vi "bin_without_level_with_enable_final.vi"() -> ()   [LabVIEW 2022 SP3]
uses:
  <vilib>/DAQmx/read.llb/DAQmx Read (Analog DBL 1Chan 1Samp).vi
  <vilib>/DAQmx/read.llb/DAQmx Read (Digital Bool 1Line 1Point).vi
  <vilib>/DAQmx/write.llb/DAQmx Write (Digital Bool 1Line 1Point).vi
  <vilib>/DAQmx/write.llb/DAQmx Write (Analog DBL 1Chan 1Samp).vi
  <vilib>/DAQmx/create/channels.llb/DAQmx Create Channel (DO-Digital Output).vi
  <vilib>/DAQmx/create/channels.llb/DAQmx Create Channel (DI-Digital Input).vi
  <vilib>/DAQmx/create/channels.llb/DAQmx Create Channel (AI-Voltage-Basic).vi
  <vilib>/DAQmx/create/channels.llb/DAQmx Create Channel (AO-Voltage-Basic).vi
  <vilib>/DAQmx/miscellaneous.llb/DAQmx Fill In Error Info.vi
panel:
  out "Boolean":bool
  out "Numeric 3":dbl format="%#_3g"
  in  "Numeric 2":dbl
  in  "Numeric":dbl
  out "String":string
  out "Weight":dbl
  in  "Linear Actuator for Plastic":tag
  in  "Linear Actuator for Plastic":tag
  in  "Linear actuator for glass":tag
  in  "Linear actuator for glass":tag
  in  "Load cell":tag
  in  "Induction proximity Sensor":tag
  in  "Linear Actuator for metal":tag
  in  "Linear Actuator for metal":tag
  in  "Exit":bool
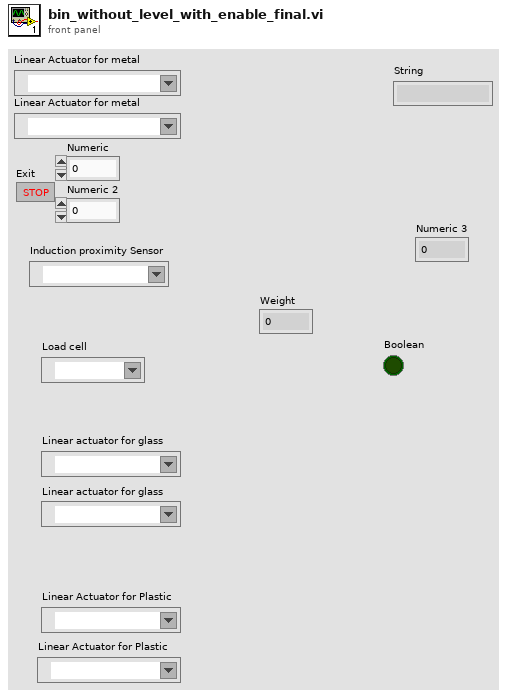
[diagram p1: front panel]
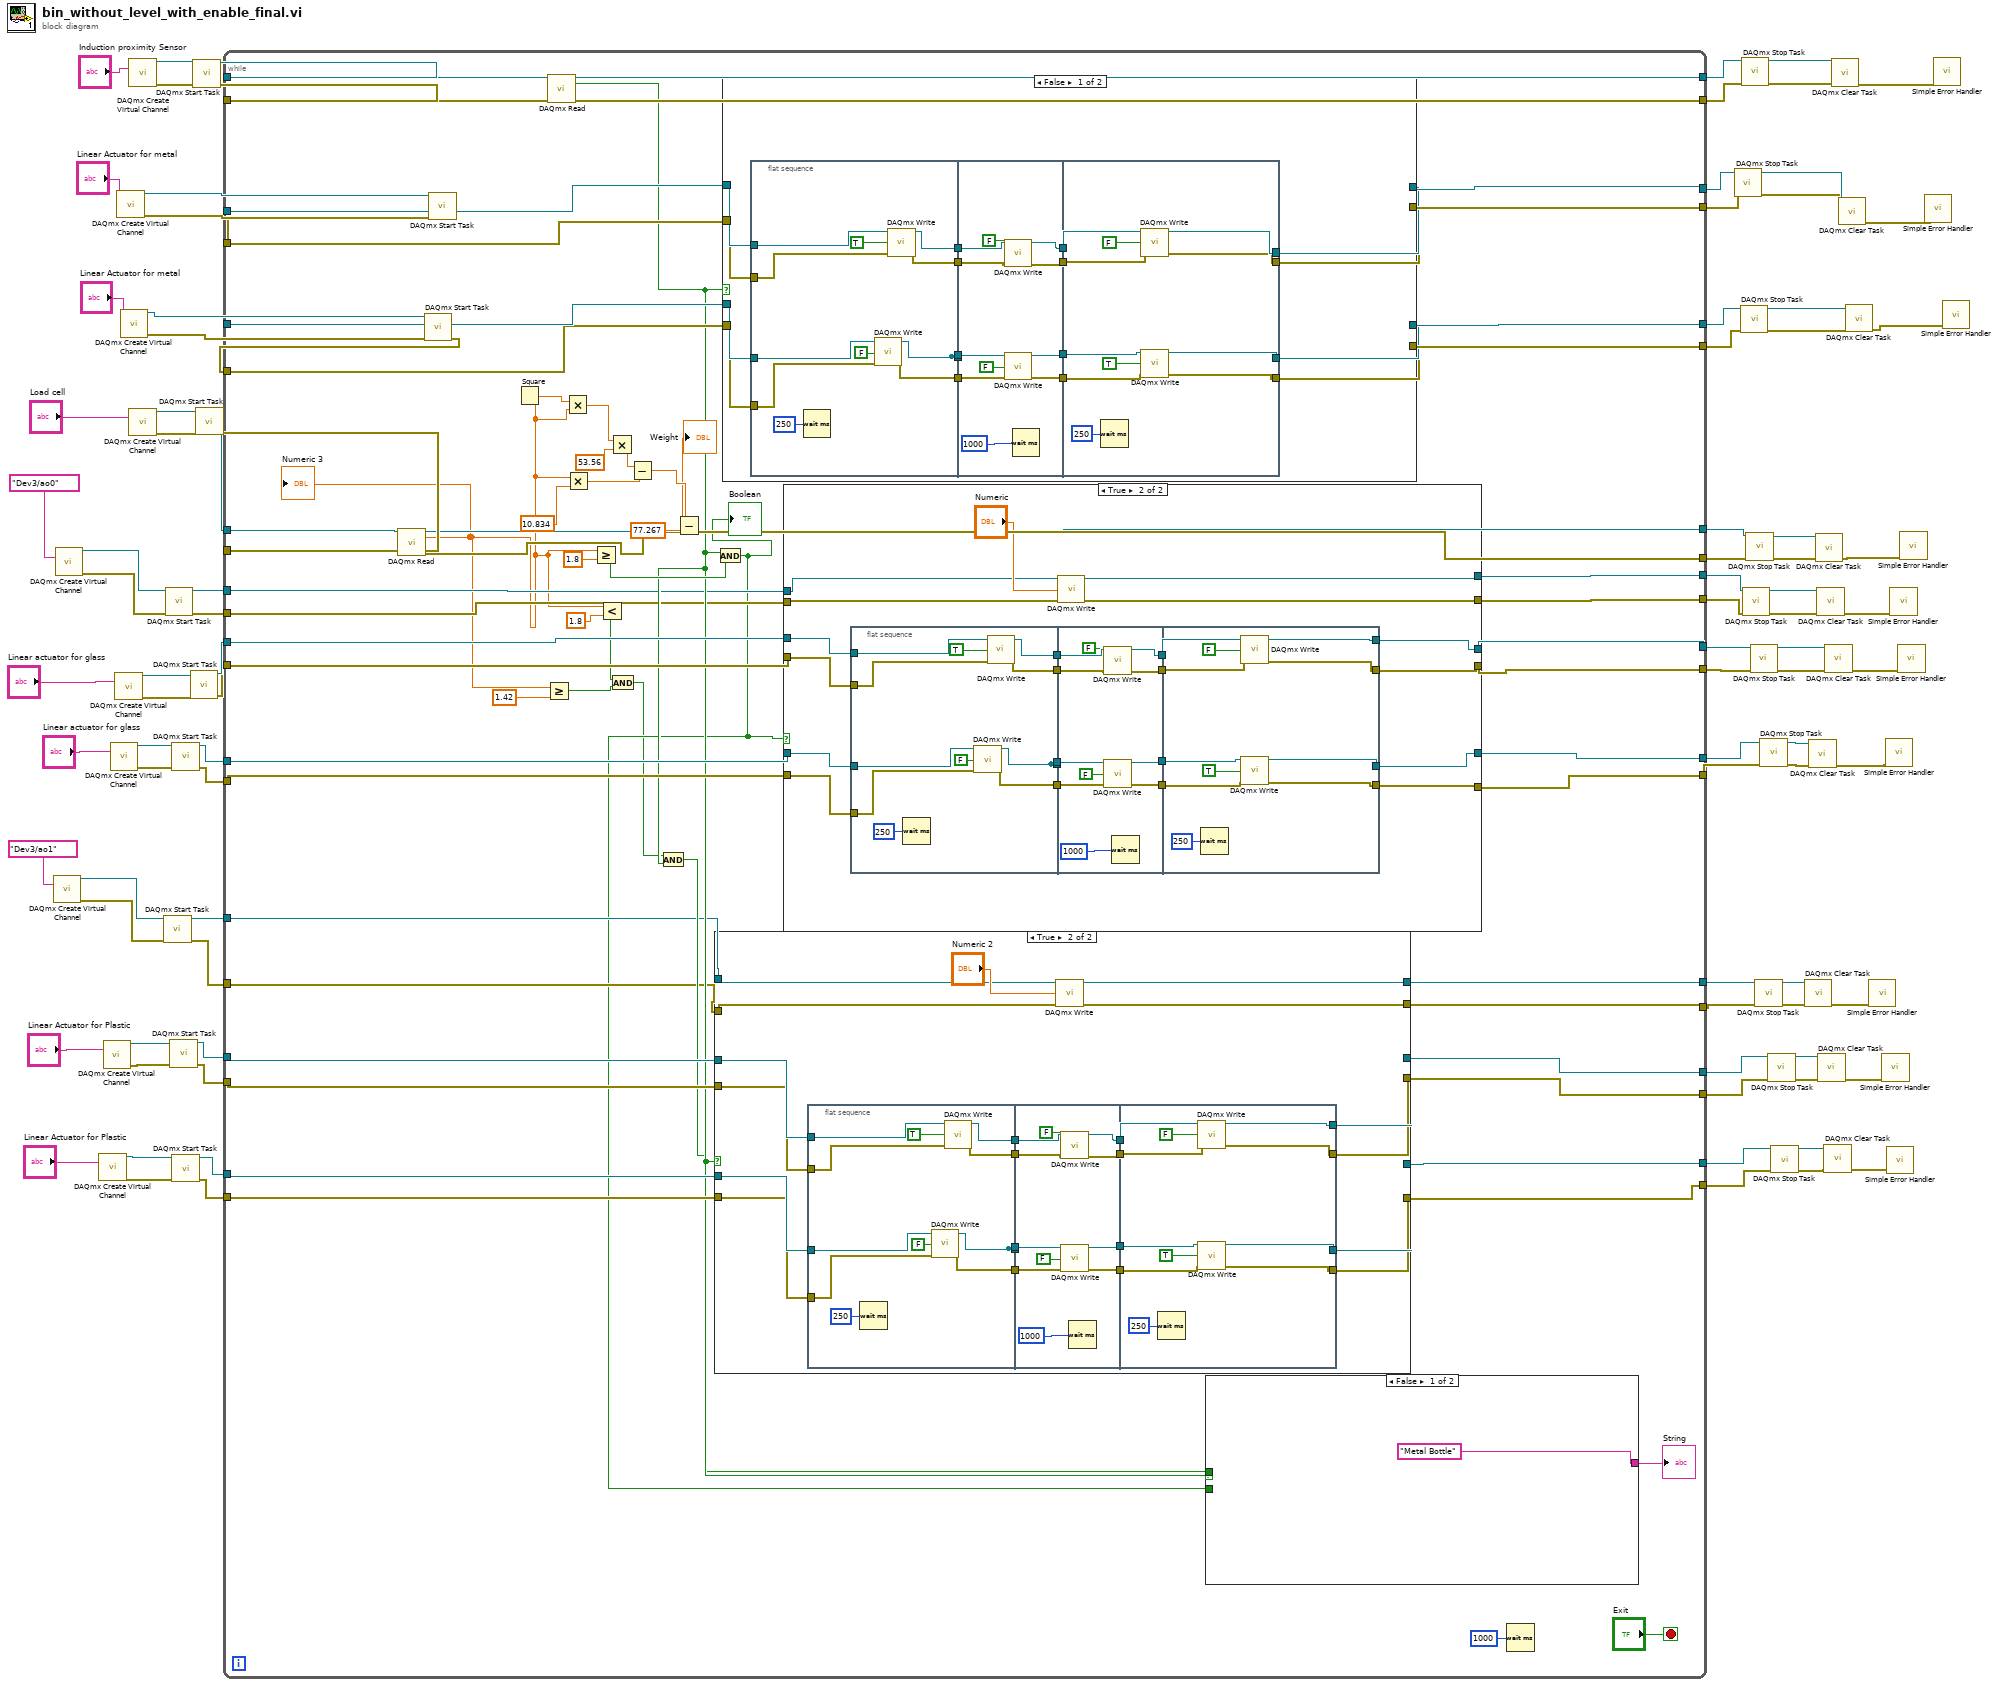
[diagram p0: block diagram]
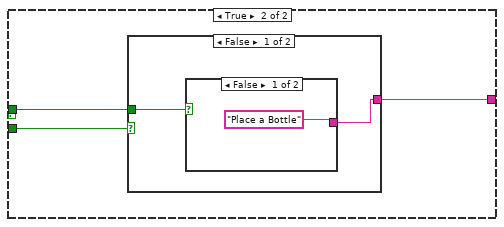
[diagram p2: hidden frame]
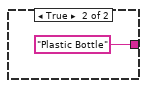
[diagram p3: hidden frame]
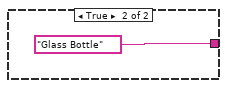
[diagram p4: hidden frame]
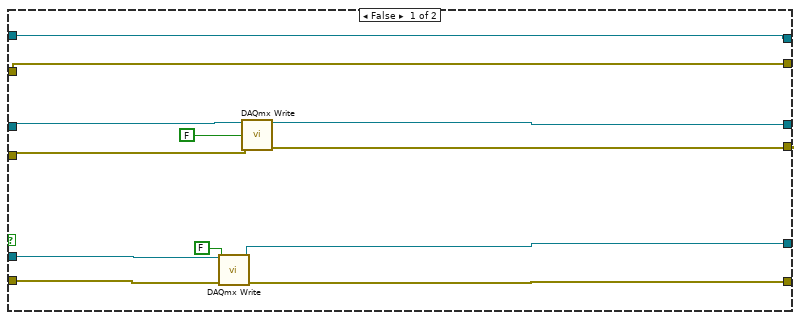
[diagram p5: hidden frame]
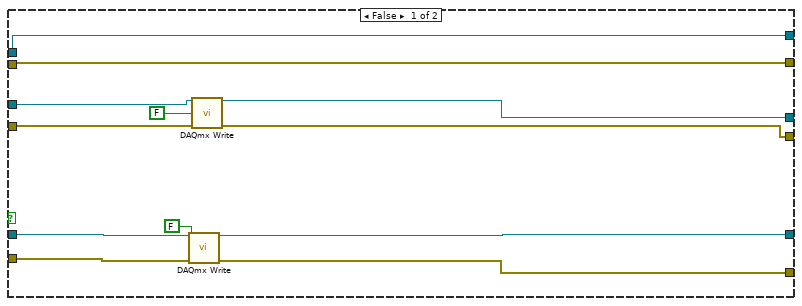
[diagram p6: hidden frame]
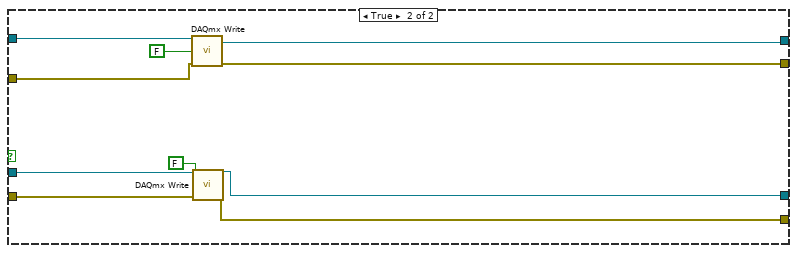
[diagram p7: hidden frame]
diagram:
  n1 = call-poly <vilib>:"DAQmx Create Virtual Channel.vi"("physical channels"=tag "Dev3/ao1") -> ("task out"=w14:refnum<k21>, "error out"=w13:errorcluster)  [unwired: 13 in]
  n2 = call-poly <vilib>:"DAQmx Create Virtual Channel.vi"("physical channels"=tag "Dev3/ao0") -> ("task out"=w19:refnum<k21>, "error out"=w18:errorcluster)  [unwired: 13 in]
  n3 = call-poly <vilib>:"DAQmx Create Virtual Channel.vi"("lines"="Linear Actuator for Plastic") -> ("task out"=w39:refnum<k21>, "error out"=w38:errorcluster)  [unwired: 13 in]
  n4 = call-poly <vilib>:"DAQmx Create Virtual Channel.vi"("lines"="Linear Actuator for Plastic") -> ("task out"=w43:refnum<k21>, "error out"=w42:errorcluster)  [unwired: 13 in]
  n5 = call-poly <vilib>:"DAQmx Create Virtual Channel.vi"("lines"="Linear actuator for glass") -> ("task out"=w59:refnum<k21>, "error out"=w58:errorcluster)  [unwired: 13 in]
  n6 = call-poly <vilib>:"DAQmx Create Virtual Channel.vi"("lines"="Linear actuator for glass") -> ("task out"=w65:refnum<k21>, "error out"=w64:errorcluster)  [unwired: 13 in]
  n7 = call-poly <vilib>:"DAQmx Create Virtual Channel.vi"("lines"="Linear Actuator for metal") -> ("task out"=w86:refnum<k21>, "error out"=w85:errorcluster)  [unwired: 13 in]
  n8 = call-poly <vilib>:"DAQmx Create Virtual Channel.vi"("lines"="Linear Actuator for metal") -> ("task out"=w90:refnum<k21>, "error out"=w89:errorcluster)  [unwired: 13 in]
  n9 = call-poly <vilib>:"DAQmx Create Virtual Channel.vi"("lines"="Induction proximity Sensor") -> ("task out"=w79:refnum<k21>, "error out"=w78:errorcluster)  [unwired: 13 in]
  n10 = call-poly <vilib>:"DAQmx Create Virtual Channel.vi"("physical channels"="Load cell") -> ("task out"=w70:refnum<k21>, "error out"=w67:errorcluster)  [unwired: 13 in]
  n11 = call <vilib>:"DAQmx Start Task.vi"("task/channels in"=w14, "error in"=w13) -> ("task out"=w12:refnum<k21>, "error out"=w11:errorcluster)  [unwired: 12 in]
  n12 = call <vilib>:"DAQmx Start Task.vi"("task/channels in"=w19, "error in"=w18) -> ("task out"=w17:refnum<k21>, "error out"=w16:errorcluster)  [unwired: 12 in]
  n13 = call <vilib>:"DAQmx Start Task.vi"("task/channels in"=w43, "error in"=w42) -> ("task out"=w41:refnum<k21>, "error out"=w40:errorcluster)  [unwired: 12 in]
  n14 = call <vilib>:"DAQmx Start Task.vi"("task/channels in"=w59, "error in"=w58) -> ("task out"=w57:refnum<k21>, "error out"=w56:errorcluster)  [unwired: 12 in]
  n15 = call <vilib>:"DAQmx Start Task.vi"("task/channels in"=w39, "error in"=w38) -> ("task out"=w37:refnum<k21>, "error out"=w36:errorcluster)  [unwired: 12 in]
  n16 = call <vilib>:"DAQmx Start Task.vi"("task/channels in"=w65, "error in"=w64) -> ("task out"=w63:refnum<k21>, "error out"=w62:errorcluster)  [unwired: 12 in]
  n17 = call <vilib>:"DAQmx Start Task.vi"("task/channels in"=w79, "error in"=w78) -> ("task out"=w77:refnum<k21>, "error out"=w76:errorcluster)  [unwired: 12 in]
  n18 = call <vilib>:"DAQmx Start Task.vi"("task/channels in"=w70, "error in"=w67) -> ("task out"=w69:refnum<k21>, "error out"=w68:errorcluster)  [unwired: 12 in]
  n19 = call <vilib>:"DAQmx Start Task.vi"("task/channels in"=w90, "error in"=w89) -> ("task out"=w88:refnum<k21>, "error out"=w87:errorcluster)  [unwired: 12 in]
  n20 = call <vilib>:"DAQmx Start Task.vi"("task/channels in"=w86, "error in"=w85) -> ("task out"=w84:refnum<k21>, "error out"=w83:errorcluster)  [unwired: 12 in]
  n21 = while {
    tunnel: w88 -> [w163]
    tunnel: w87 -> [w162]
    tunnel: w84 -> [w161]
    tunnel: w83 -> [w160]
    tunnel: [w159] -> w98
    tunnel: [w158] -> w97
    tunnel: [w157] -> w96
    tunnel: [w156] -> w95
    tunnel: w77 -> [w154]
    tunnel: w76 -> [w153]
    tunnel: [w152] -> w72
    tunnel: [w151] -> w71
    tunnel: w69 -> [w150]
    tunnel: w68 -> [w149]
    tunnel: w63 -> [w147]
    tunnel: w62 -> [w146]
    tunnel: w57 -> [w145]
    tunnel: w56 -> [w144]
    tunnel: [w143] -> w55
    tunnel: [w140] -> w54
    tunnel: [w142] -> w48
    tunnel: [w141] -> w47
    tunnel: w41 -> [w138]
    tunnel: w40 -> [w137]
    tunnel: w37 -> [w136]
    tunnel: w36 -> [w135]
    tunnel: [w134] -> w29
    tunnel: [w133] -> w28
    tunnel: [w132] -> w27
    tunnel: [w131] -> w26
    tunnel: [w118] -> w22
    tunnel: [w117] -> w21
    tunnel: w17 -> [w114]
    tunnel: w16 -> [w113]
    tunnel: w12 -> [w112]
    tunnel: w11 -> [w111]
    tunnel: [w110] -> w7
    tunnel: [w109] -> w6
    tunnel: [w107] -> w2
    tunnel: [w108] -> w1
    stop <- "Exit" stop-if-true
    n22 = call-poly <vilib>:"DAQmx Read.vi"("task/channels in"=w150, "error in"=w149) -> ("task out"=w117:refnum<k21>, "data"=w104:dbl, "error out"=w118:errorcluster)  [unwired: 11 in]
    "Numeric 3" <- w104
    n23 = Square(x=w104) -> (x^2=w123:dbl)
    n24 = Greater Or Equal?(x=w104, y=1.42) -> (x >= y?=w102:bool)
    n25 = call-poly <vilib>:"DAQmx Read.vi"("task/channels in"=w154, "error in"=w153) -> ("task out"=w151:refnum<k21>, "data"=w116:bool, "error out"=w152:errorcluster)  [unwired: 11 in]
    n26 = Multiply(x=w123, y=w104) -> (x*y=w122:dbl)
    n27 = Multiply(x=w104, y=10.834) -> (x*y=w127:dbl)
    n28 = Greater Or Equal?(x=w104, y=1.8) -> (x >= y?=w148:bool)
    n29 = Less?(x=w104, y=1.8) -> (x < y?=w103:bool)
    n30 = Multiply(x=w122, y=53.56) -> (x*y=w129:dbl)
    n31 = And(x=w103, y=w102) -> (x .and. y?=w101:bool)
    n32 = Subtract(x=w129, y=w127) -> (x-y=w126:dbl)
    n33 = And(x=w101, y=w116) -> (x .and. y?=w115:bool)
    n34 = Subtract(x=w126, y=77.267) -> (x-y=→"Weight":dbl)
    n35 = case shown="True" w115 {
      tunnel: w136 -> [w184 w206]
      tunnel: w135 -> [w177 w205]
      tunnel: w138 -> [w179 w204]
      tunnel: w137 -> [w178 w203]
      tunnel: [w183 w193] -> w131
      tunnel: [w182 w192] -> w132
      tunnel: [w181 w191] -> w134
      tunnel: [w180 w190] -> w133
      tunnel: w112 -> [w174 w187]
      tunnel: w111 -> [w173 w188]
      tunnel: [w174 w186] -> w107
      tunnel: [w173 w185] -> w108
      frame False {
        n36 = call-poly <vilib>:"DAQmx Write.vi"("task/channels in"=w184, "data"=FALSE, "error in"=w177) -> ("task out"=w181:refnum<k21>, "error out"=w180:errorcluster)  [unwired: 10 in, 1 out]
        n37 = call-poly <vilib>:"DAQmx Write.vi"("task/channels in"=w179, "data"=FALSE, "error in"=w178) -> ("task out"=w183:refnum<k21>, "error out"=w182:errorcluster)  [unwired: 10 in, 1 out]
      }
      frame True {
        n38 = flat-sequence {
          tunnel: w206 -> [w217]
          tunnel: w205 -> [w216]
          tunnel: w204 -> [w215]
          tunnel: w203 -> [w214]
          tunnel: [w211] -> w202
          tunnel: [w210] -> w200
          tunnel: [w207] -> w198
          tunnel: [w209] -> w196
          tunnel: [w207] -> w194
          tunnel: w202 -> [w228]
          tunnel: [w227] -> w201
          tunnel: w200 -> [w226]
          tunnel: [w225] -> w199
          tunnel: w198 -> [_]
          tunnel: [w222] -> w197
          tunnel: w196 -> [w220]
          tunnel: [w223] -> w195
          tunnel: w194 -> [w221]
          tunnel: [w233] -> w191
          tunnel: [w234] -> w192
          tunnel: [w235] -> w193
          tunnel: w201 -> [w239]
          tunnel: w199 -> [w238]
          tunnel: w197 -> [w237]
          tunnel: w195 -> [w236]
          tunnel: [w232] -> w190
          frame #0 {
            n39 = Wait (ms)(milliseconds to wait=u32 250) -> ()  [unwired: 1 out]
            n40 = call-poly <vilib>:"DAQmx Write.vi"("task/channels in"=w217, "data"=FALSE, "error in"=w216) -> ("task out"=w207:refnum<k21>, "error out"=w209:errorcluster)  [unwired: 10 in, 1 out]
            n41 = call-poly <vilib>:"DAQmx Write.vi"("task/channels in"=w215, "data"=TRUE, "error in"=w214) -> ("task out"=w211:refnum<k21>, "error out"=w210:errorcluster)  [unwired: 10 in, 1 out]
          }
          frame #1 {
            n42 = call-poly <vilib>:"DAQmx Write.vi"("task/channels in"=w228, "data"=FALSE, "error in"=w226) -> ("task out"=w227:refnum<k21>, "error out"=w225:errorcluster)  [unwired: 10 in, 1 out]
            n43 = call-poly <vilib>:"DAQmx Write.vi"("task/channels in"=w221, "data"=FALSE, "error in"=w220) -> ("task out"=w222:refnum<k21>, "error out"=w223:errorcluster)  [unwired: 10 in, 1 out]
            n44 = Wait (ms)(milliseconds to wait=u32 1000 ("millisecond timer value")) -> ()  [unwired: 1 out]
          }
          frame #2 {
            n45 = Wait (ms)(milliseconds to wait=u32 250) -> ()  [unwired: 1 out]
            n46 = call-poly <vilib>:"DAQmx Write.vi"("task/channels in"=w239, "data"=FALSE, "error in"=w238) -> ("task out"=w235:refnum<k21>, "error out"=w234:errorcluster)  [unwired: 10 in, 1 out]
            n47 = call-poly <vilib>:"DAQmx Write.vi"("task/channels in"=w237, "data"=TRUE, "error in"=w236) -> ("task out"=w233:refnum<k21>, "error out"=w232:errorcluster)  [unwired: 10 in, 1 out]
          }
        }
        n48 = call-poly <vilib>:"DAQmx Write.vi"("task/channels in"=w187, "data"="Numeric 2", "error in"=w188) -> ("task out"=w186:refnum<k21>, "error out"=w185:errorcluster)  [unwired: 10 in, 1 out]
      }
    }
    n49 = And(x=w116, y=w148) -> (x .and. y?=w106:bool)
    "Boolean" <- w106
    n50 = case shown="False" w116 {
      tunnel: w163 -> [w323 w364]
      tunnel: w162 -> [w322 w363]
      tunnel: w161 -> [w321 w366]
      tunnel: w160 -> [w320 w365]
      tunnel: [w319 w360] -> w159
      tunnel: [w318 w359] -> w158
      tunnel: [w317 w358] -> w157
      tunnel: [w316 w357] -> w156
      frame False {
        n51 = flat-sequence {
          tunnel: w323 -> [w334]
          tunnel: w322 -> [w333]
          tunnel: w321 -> [w332]
          tunnel: w320 -> [w331]
          tunnel: [w328] -> w315
          tunnel: [w327] -> w313
          tunnel: [w324] -> w311
          tunnel: [w326] -> w309
          tunnel: [w324] -> w307
          tunnel: w315 -> [w345]
          tunnel: [w344] -> w314
          tunnel: w313 -> [w343]
          tunnel: [w342] -> w312
          tunnel: w311 -> [_]
          tunnel: [w339] -> w310
          tunnel: w309 -> [w337]
          tunnel: [w340] -> w308
          tunnel: w307 -> [w338]
          tunnel: [w350] -> w317
          tunnel: [w351] -> w318
          tunnel: [w352] -> w319
          tunnel: w314 -> [w356]
          tunnel: w312 -> [w355]
          tunnel: w310 -> [w354]
          tunnel: w308 -> [w353]
          tunnel: [w349] -> w316
          frame #0 {
            n52 = Wait (ms)(milliseconds to wait=u32 250) -> ()  [unwired: 1 out]
            n53 = call-poly <vilib>:"DAQmx Write.vi"("task/channels in"=w334, "data"=FALSE, "error in"=w333) -> ("task out"=w324:refnum<k21>, "error out"=w326:errorcluster)  [unwired: 10 in, 1 out]
            n54 = call-poly <vilib>:"DAQmx Write.vi"("task/channels in"=w332, "data"=TRUE, "error in"=w331) -> ("task out"=w328:refnum<k21>, "error out"=w327:errorcluster)  [unwired: 10 in, 1 out]
          }
          frame #1 {
            n55 = call-poly <vilib>:"DAQmx Write.vi"("task/channels in"=w345, "data"=FALSE, "error in"=w343) -> ("task out"=w344:refnum<k21>, "error out"=w342:errorcluster)  [unwired: 10 in, 1 out]
            n56 = call-poly <vilib>:"DAQmx Write.vi"("task/channels in"=w338, "data"=FALSE, "error in"=w337) -> ("task out"=w339:refnum<k21>, "error out"=w340:errorcluster)  [unwired: 10 in, 1 out]
            n57 = Wait (ms)(milliseconds to wait=u32 1000 ("millisecond timer value")) -> ()  [unwired: 1 out]
          }
          frame #2 {
            n58 = Wait (ms)(milliseconds to wait=u32 250) -> ()  [unwired: 1 out]
            n59 = call-poly <vilib>:"DAQmx Write.vi"("task/channels in"=w356, "data"=FALSE, "error in"=w355) -> ("task out"=w352:refnum<k21>, "error out"=w351:errorcluster)  [unwired: 10 in, 1 out]
            n60 = call-poly <vilib>:"DAQmx Write.vi"("task/channels in"=w354, "data"=TRUE, "error in"=w353) -> ("task out"=w350:refnum<k21>, "error out"=w349:errorcluster)  [unwired: 10 in, 1 out]
          }
        }
      }
      frame True {
        n61 = call-poly <vilib>:"DAQmx Write.vi"("task/channels in"=w366, "data"=FALSE, "error in"=w365) -> ("task out"=w360:refnum<k21>, "error out"=w359:errorcluster)  [unwired: 10 in, 1 out]
        n62 = call-poly <vilib>:"DAQmx Write.vi"("task/channels in"=w364, "data"=FALSE, "error in"=w363) -> ("task out"=w358:refnum<k21>, "error out"=w357:errorcluster)  [unwired: 10 in, 1 out]
      }
    }
    n63 = case shown="True" w106 {
      tunnel: w145 -> [w251 w273]
      tunnel: w144 -> [w244 w272]
      tunnel: w147 -> [w246 w271]
      tunnel: w146 -> [w245 w270]
      tunnel: [w250 w260] -> w143
      tunnel: [w249 w259] -> w140
      tunnel: [w248 w258] -> w142
      tunnel: [w247 w257] -> w141
      tunnel: w114 -> [w241 w255]
      tunnel: w113 -> [w240 w254]
      tunnel: [w241 w253] -> w110
      tunnel: [w240 w252] -> w109
      frame False {
        n64 = call-poly <vilib>:"DAQmx Write.vi"("task/channels in"=w251, "data"=FALSE, "error in"=w244) -> ("task out"=w248:refnum<k21>, "error out"=w247:errorcluster)  [unwired: 10 in, 1 out]
        n65 = call-poly <vilib>:"DAQmx Write.vi"("task/channels in"=w246, "data"=FALSE, "error in"=w245) -> ("task out"=w250:refnum<k21>, "error out"=w249:errorcluster)  [unwired: 10 in, 1 out]
      }
      frame True {
        n66 = flat-sequence {
          tunnel: w273 -> [w284]
          tunnel: w272 -> [w283]
          tunnel: w271 -> [w282]
          tunnel: w270 -> [w281]
          tunnel: [w278] -> w269
          tunnel: [w277] -> w267
          tunnel: [w274] -> w265
          tunnel: [w276] -> w263
          tunnel: [w274] -> w261
          tunnel: w269 -> [w295]
          tunnel: [w294] -> w268
          tunnel: w267 -> [w293]
          tunnel: [w292] -> w266
          tunnel: w265 -> [_]
          tunnel: [w289] -> w264
          tunnel: w263 -> [w287]
          tunnel: [w290] -> w262
          tunnel: w261 -> [w288]
          tunnel: [w300] -> w258
          tunnel: [w301] -> w259
          tunnel: [w302] -> w260
          tunnel: w268 -> [w306]
          tunnel: w266 -> [w305]
          tunnel: w264 -> [w304]
          tunnel: w262 -> [w303]
          tunnel: [w299] -> w257
          frame #0 {
            n67 = Wait (ms)(milliseconds to wait=u32 250) -> ()  [unwired: 1 out]
            n68 = call-poly <vilib>:"DAQmx Write.vi"("task/channels in"=w284, "data"=FALSE, "error in"=w283) -> ("task out"=w274:refnum<k21>, "error out"=w276:errorcluster)  [unwired: 10 in, 1 out]
            n69 = call-poly <vilib>:"DAQmx Write.vi"("task/channels in"=w282, "data"=TRUE, "error in"=w281) -> ("task out"=w278:refnum<k21>, "error out"=w277:errorcluster)  [unwired: 10 in, 1 out]
          }
          frame #1 {
            n70 = call-poly <vilib>:"DAQmx Write.vi"("task/channels in"=w295, "data"=FALSE, "error in"=w293) -> ("task out"=w294:refnum<k21>, "error out"=w292:errorcluster)  [unwired: 10 in, 1 out]
            n71 = call-poly <vilib>:"DAQmx Write.vi"("task/channels in"=w288, "data"=FALSE, "error in"=w287) -> ("task out"=w289:refnum<k21>, "error out"=w290:errorcluster)  [unwired: 10 in, 1 out]
            n72 = Wait (ms)(milliseconds to wait=u32 1000 ("millisecond timer value")) -> ()  [unwired: 1 out]
          }
          frame #2 {
            n73 = Wait (ms)(milliseconds to wait=u32 250) -> ()  [unwired: 1 out]
            n74 = call-poly <vilib>:"DAQmx Write.vi"("task/channels in"=w306, "data"=FALSE, "error in"=w305) -> ("task out"=w302:refnum<k21>, "error out"=w301:errorcluster)  [unwired: 10 in, 1 out]
            n75 = call-poly <vilib>:"DAQmx Write.vi"("task/channels in"=w304, "data"=TRUE, "error in"=w303) -> ("task out"=w300:refnum<k21>, "error out"=w299:errorcluster)  [unwired: 10 in, 1 out]
          }
        }
        n76 = call-poly <vilib>:"DAQmx Write.vi"("task/channels in"=w255, "data"="Numeric", "error in"=w254) -> ("task out"=w253:refnum<k21>, "error out"=w252:errorcluster)  [unwired: 10 in, 1 out]
      }
    }
    n77 = case shown="False" w116 {
      tunnel: ["Metal Bottle" w167] -> w119
      tunnel: w106 -> [_ w166]
      tunnel: w115 -> [_ w165]
      frame False {
      }
      frame True {
        n78 = case shown="False" w166 {
          tunnel: [w169 "Glass Bottle"] -> w167
          tunnel: w165 -> [w168 _]
          frame False {
            n79 = case shown="False" w168 {
              tunnel: ["Place a Bottle" "Plastic Bottle"] -> w169
              frame False {
              }
              frame True {
              }
            }
          }
          frame True {
          }
        }
      }
    }
    "String" <- w119
    n80 = Wait (ms)(milliseconds to wait=u32 1000) -> ()  [unwired: 1 out]
  }
  n81 = call <vilib>:"DAQmx Stop Task.vi"("task/channels in"=w98, "error in"=w97) -> ("task out"=w94:refnum<k21>, "error out"=w93:errorcluster)  [unwired: 12 in]
  n82 = call <vilib>:"DAQmx Stop Task.vi"("task/channels in"=w96, "error in"=w95) -> ("task out"=w92:refnum<k21>, "error out"=w91:errorcluster)  [unwired: 12 in]
  n83 = call <vilib>:"DAQmx Stop Task.vi"("task/channels in"=w71, "error in"=w72) -> ("task out"=w75:refnum<k21>, "error out"=w74:errorcluster)  [unwired: 12 in]
  n84 = call <vilib>:"DAQmx Stop Task.vi"("task/channels in"=w7, "error in"=w6) -> ("task out"=w10:refnum<k21>, "error out"=w9:errorcluster)  [unwired: 12 in]
  n85 = call <vilib>:"DAQmx Stop Task.vi"("task/channels in"=w21, "error in"=w22) -> ("task out"=w23:refnum<k21>, "error out"=w24:errorcluster)  [unwired: 12 in]
  n86 = call <vilib>:"DAQmx Stop Task.vi"("task/channels in"=w55, "error in"=w54) -> ("task out"=w53:refnum<k21>, "error out"=w52:errorcluster)  [unwired: 12 in]
  n87 = call <vilib>:"DAQmx Stop Task.vi"("task/channels in"=w2, "error in"=w1) -> ("task out"=w5:refnum<k21>, "error out"=w4:errorcluster)  [unwired: 12 in]
  n88 = call <vilib>:"DAQmx Stop Task.vi"("task/channels in"=w48, "error in"=w47) -> ("task out"=w50:refnum<k21>, "error out"=w49:errorcluster)  [unwired: 12 in]
  n89 = call <vilib>:"DAQmx Stop Task.vi"("task/channels in"=w26, "error in"=w27) -> ("task out"=w35:refnum<k21>, "error out"=w34:errorcluster)  [unwired: 12 in]
  n90 = call <vilib>:"DAQmx Stop Task.vi"("task/channels in"=w29, "error in"=w28) -> ("task out"=w31:refnum<k21>, "error out"=w30:errorcluster)  [unwired: 12 in]
  n91 = call <vilib>:"DAQmx Clear Task.vi"("task in"=w5, "error in"=w4) -> ("error out"=w3:errorcluster)  [unwired: 13 in]
  n92 = call <vilib>:"DAQmx Clear Task.vi"("task in"=w50, "error in"=w49) -> ("error out"=w46:errorcluster)  [unwired: 13 in]
  n93 = call <vilib>:"DAQmx Clear Task.vi"("task in"=w23, "error in"=w24) -> ("error out"=w25:errorcluster)  [unwired: 13 in]
  n94 = call <vilib>:"DAQmx Clear Task.vi"("task in"=w10, "error in"=w9) -> ("error out"=w8:errorcluster)  [unwired: 13 in]
  n95 = call <vilib>:"DAQmx Clear Task.vi"("task in"=w35, "error in"=w34) -> ("error out"=w33:errorcluster)  [unwired: 13 in]
  n96 = call <vilib>:"DAQmx Clear Task.vi"("task in"=w31, "error in"=w30) -> ("error out"=w32:errorcluster)  [unwired: 13 in]
  n97 = call <vilib>:"DAQmx Clear Task.vi"("task in"=w53, "error in"=w52) -> ("error out"=w51:errorcluster)  [unwired: 13 in]
  n98 = call <vilib>:"DAQmx Clear Task.vi"("task in"=w75, "error in"=w74) -> ("error out"=w73:errorcluster)  [unwired: 13 in]
  n99 = call <vilib>:"DAQmx Clear Task.vi"("task in"=w94, "error in"=w93) -> ("error out"=w100:errorcluster)  [unwired: 13 in]
  n100 = call <vilib>:"DAQmx Clear Task.vi"("task in"=w92, "error in"=w91) -> ("error out"=w99:errorcluster)  [unwired: 13 in]
  n101 = call <vilib>:"Simple Error Handler.vi"("error in (no error)"=w3) -> ()  [unwired: 4 in, 5 out]
  n102 = call <vilib>:"Simple Error Handler.vi"("error in (no error)"=w33) -> ()  [unwired: 4 in, 5 out]
  n103 = call <vilib>:"Simple Error Handler.vi"("error in (no error)"=w46) -> ()  [unwired: 4 in, 5 out]
  n104 = call <vilib>:"Simple Error Handler.vi"("error in (no error)"=w32) -> ()  [unwired: 4 in, 5 out]
  n105 = call <vilib>:"Simple Error Handler.vi"("error in (no error)"=w8) -> ()  [unwired: 4 in, 5 out]
  n106 = call <vilib>:"Simple Error Handler.vi"("error in (no error)"=w51) -> ()  [unwired: 4 in, 5 out]
  n107 = call <vilib>:"Simple Error Handler.vi"("error in (no error)"=w25) -> ()  [unwired: 4 in, 5 out]
  n108 = call <vilib>:"Simple Error Handler.vi"("error in (no error)"=w100) -> ()  [unwired: 4 in, 5 out]
  n109 = call <vilib>:"Simple Error Handler.vi"("error in (no error)"=w73) -> ()  [unwired: 4 in, 5 out]
  n110 = call <vilib>:"Simple Error Handler.vi"("error in (no error)"=w99) -> ()  [unwired: 4 in, 5 out]
